vi "WUP.vi"() -> ()   [LabVIEW 2013]
uses:
  <userlib>/_OpenG.lib/array/array.llb/Index 1D Array Elements (String)__ogtk.vi
panel:
  in  "Experiment":u16(ring) items=["10TW", "test stand", "LaserUpstairs", "Staging"]
  out "clients dead":i16
  out "clients alive":i16
  in  "remote desktop":bool
  in  "Scrollbar":i32(c297)
  in  "cmd":bool
  out "Message 3":string
  in  "CMD":string
  out "error out 2":errorcluster
  in  "enter":bool
  out "elements":string[](array[string])
  in  "Listbox":i32[](listbox)
  out "output cluster":T1
  in  "ping":bool
  in  "WUP and restart":bool
  in  "stop":bool
  out "Message 2":string="\\\\192.168.10.217\\Documents\\Software\\LABVIEW\\Sven\\test\\wuInstall /search /criteria \"IsInstalled=0 and AutoSelectOnWebSites=1\""
  out "error out":errorcluster
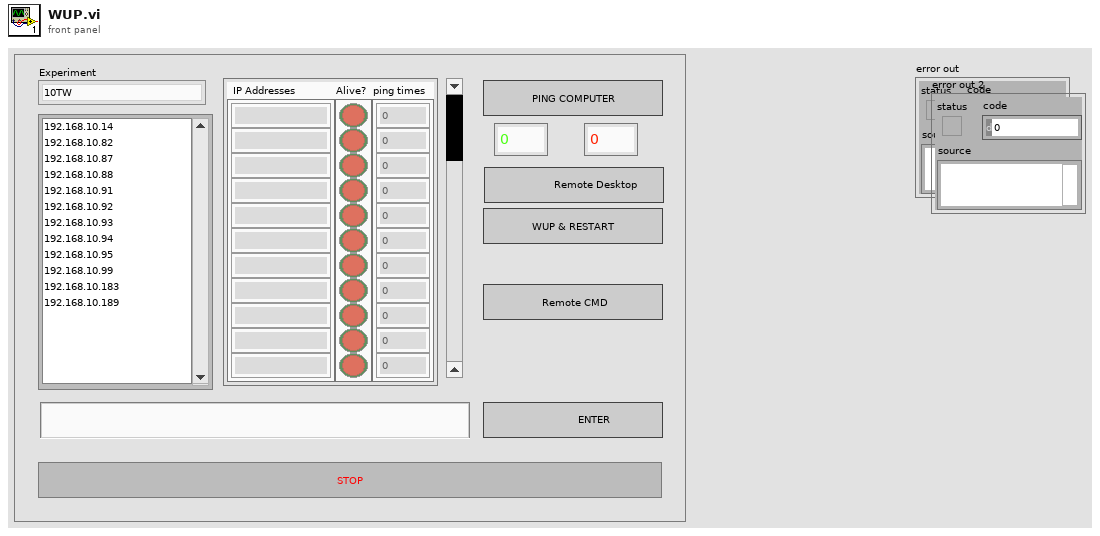
[diagram p1: front panel]
types:
  T1 = cluster{"IP Addresses ":string[], "Alive?":bool[], "ping times":u32[]}
  T2 = cluster{"elements":string[], "Awake?":bool[], "ping times [ms]":u32[]}
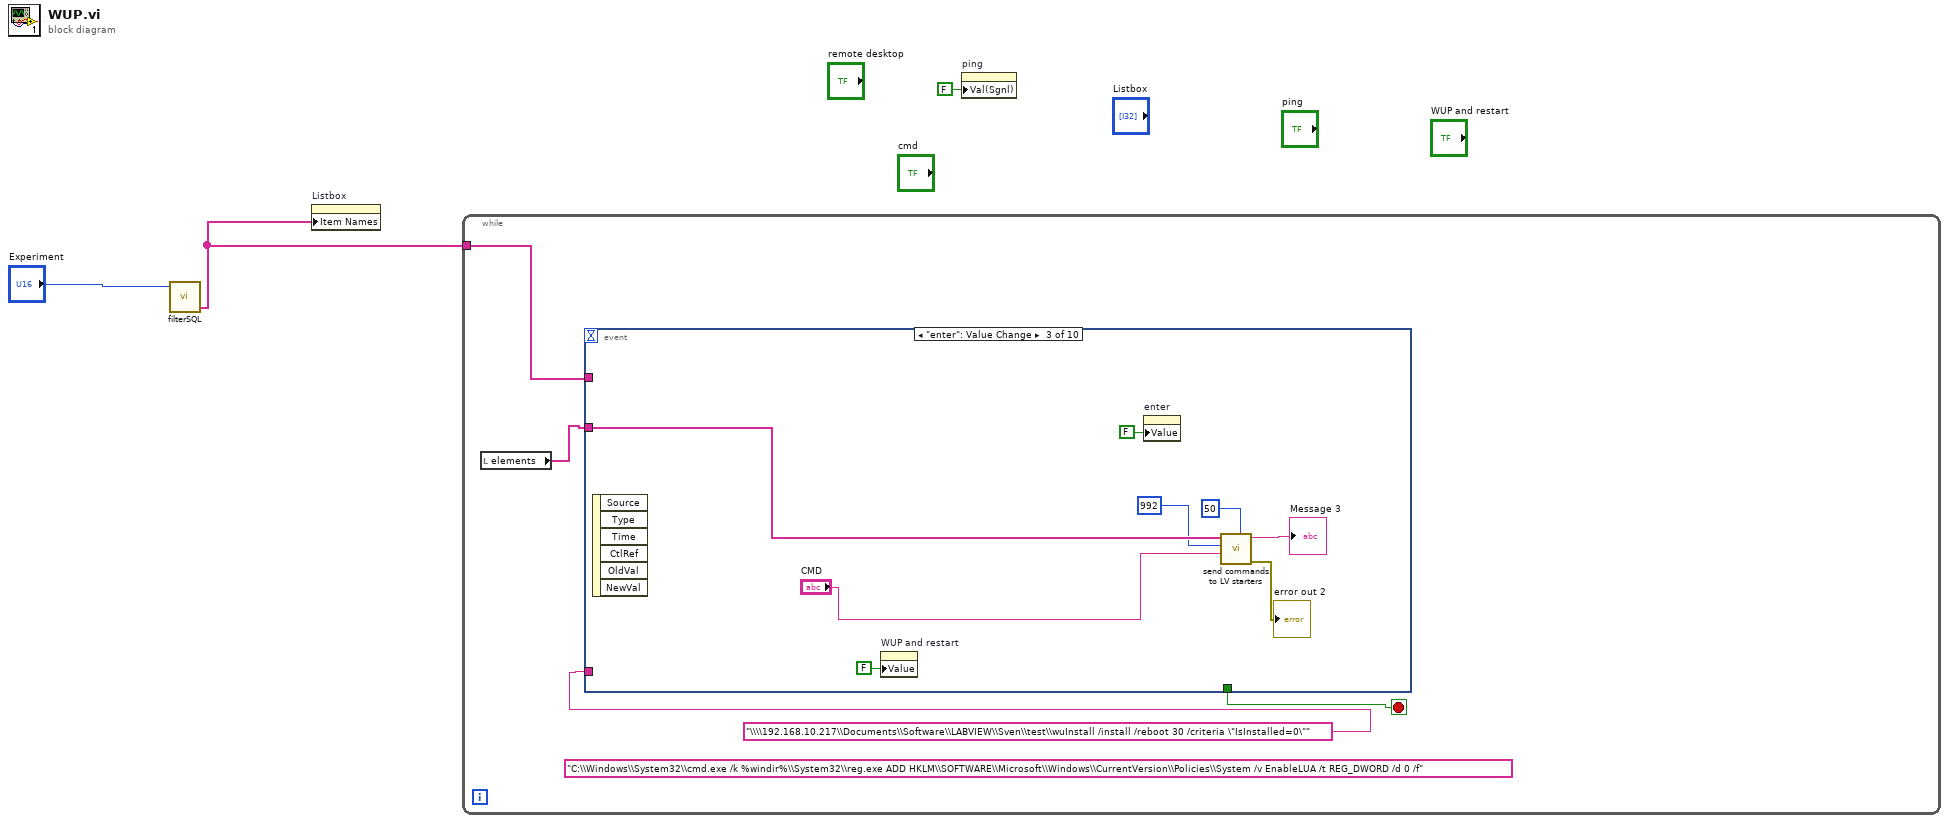
[diagram p0: block diagram]
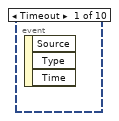
[diagram p2: hidden frame]
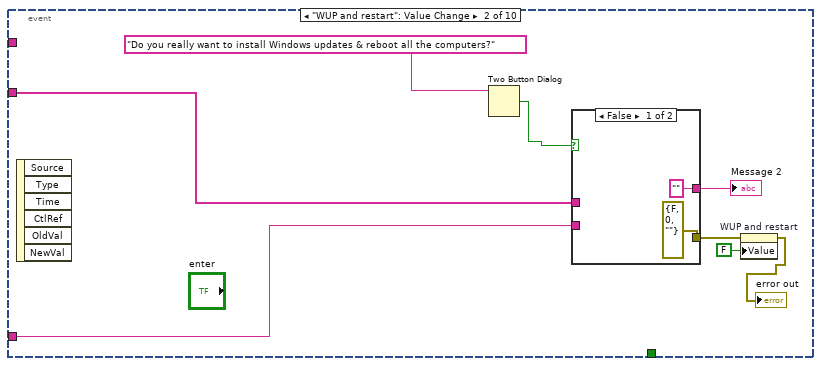
[diagram p3: hidden frame]
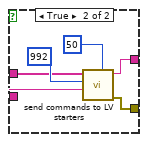
[diagram p4: hidden frame]
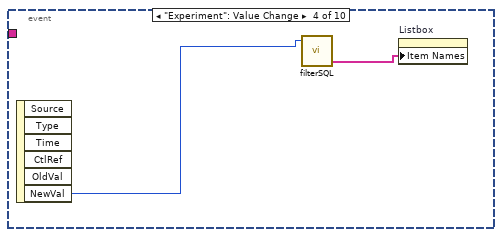
[diagram p5: hidden frame]
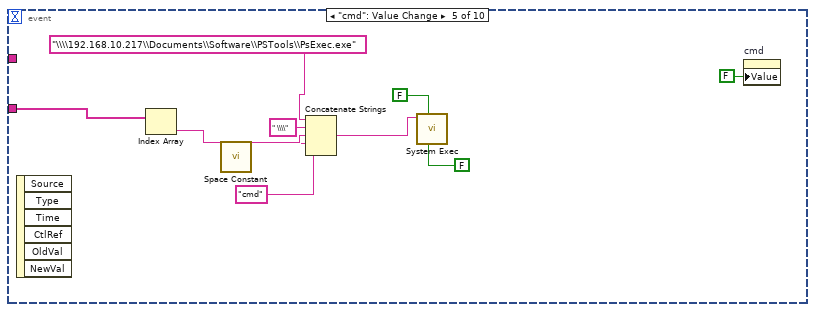
[diagram p6: hidden frame]
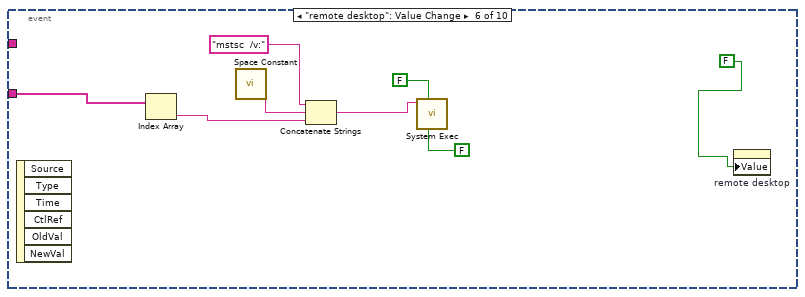
[diagram p7: hidden frame]
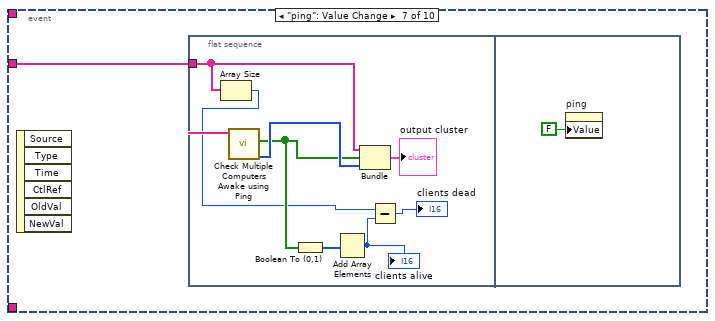
[diagram p8: hidden frame]
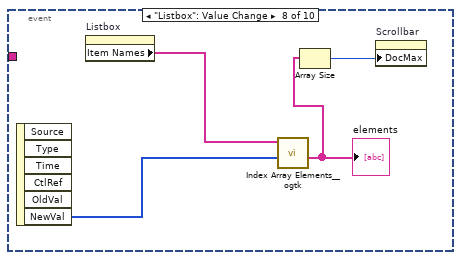
[diagram p9: hidden frame]
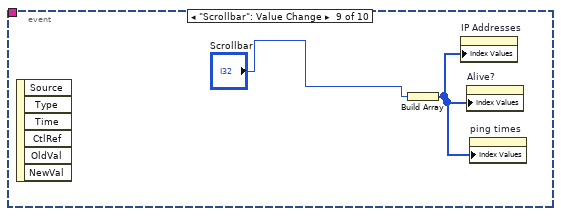
[diagram p10: hidden frame]
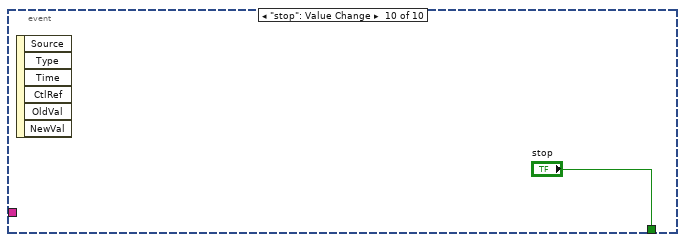
[diagram p11: hidden frame]
diagram:
  n1 = call "filterSQL.vi"("Experiment"="Experiment") -> ("filtered"=w1:string[])  [unwired: 3 in, 1 out]
  n2 = property on="Listbox" class="LstBox (strict)"("Item Names"=w1) -> ()  [unwired: 2 in, 2 out]
  n3 = while {
    tunnel: w1 -> [w6]
    stop <- w7 stop-if-true
    (unwired) "C:\\Windows\\System32\\cmd.exe /k %windir%\\System32\\reg.exe ADD HKLM\\SOFTWARE\\Microsoft\\Windows\\CurrentVersion\\Policies\\System /v EnableLUA /t REG_DWORD /d 0 /f"
    n4 = local read "elements"() -> (w4:string[])
    n5 = event shown="[2] \"enter\": Value Change" {
      selector: _ -> [_ _ _ _ _ _ _ _ _ _]
      dyn-events: _ -> [_ _ _ _ _ _ _ _ _ _]
      timeout: _ -> [_ _ _ _ _ _ _ _ _ _]
      tunnel: "\\\\192.168.10.217\\Documents\\Software\\LABVIEW\\Sven\\test\\wuInstall /install /reboot 30 /criteria \"IsInstalled=0\"" ("Message") -> [_ w15 _ _ _ _ _ _ _ _]
      tunnel: [_ _ _ _ _ _ _ _ _ "stop"] -> w7
      tunnel: w4 -> [_ w11 w30 _ w42 w51 w52 _ _ _]
      tunnel: w6 -> [_ _ _ _ _ _ _ _ _ _]
      event Timeout {
        n6 = event-data() -> ()  [unwired: 1 in, 3 out]
      }
      event "WUP and restart": Value Change {
        n7 = event-data() -> ()  [unwired: 1 in, 6 out]
        n8 = Two Button Dialog(message="Do you really want to install Windows updates & reboot all the computers?") -> (T button?=w12:bool)  [unwired: 2 in]
        n9 = case shown="False" w12 {
          tunnel: w11 -> [_ w21]
          tunnel: w15 -> [_ w20]
          tunnel: [errorcluster {"status"=FALSE, "code"=0, "source"=""} ("error out") w19] -> w10
          tunnel: ["" ("Message 2") w18] -> w8
          frame False {
          }
          frame True {
            n10 = call "send commands to LV starters.vi"("IP Addresses"=w21, "Local Port"=u16 992, "Message"=w20, "time between commands (ms)"=u32 50) -> ("Message 2"=w18:string, "error out"=w19:errorcluster)  [unwired: 4 in]
          }
        }
        "Message 2" <- w8
        n11 = property on="WUP and restart" class="Bool (strict)"(error in=w10, "Value"=FALSE ("WUP and restart")) -> (error out=→"error out":errorcluster)  [unwired: 1 in, 1 out]
      }
      event "enter": Value Change {
        n12 = event-data() -> ()  [unwired: 1 in, 6 out]
        n13 = property on="WUP and restart" class="Bool (strict)"("Value"=FALSE ("WUP and restart")) -> ()  [unwired: 2 in, 2 out]
        n14 = property on="enter" class="Bool (strict)"("Value"=FALSE ("enter")) -> ()  [unwired: 2 in, 2 out]
        n15 = call "send commands to LV starters.vi"("IP Addresses"=w30, "Local Port"=u16 992, "Message"="CMD", "time between commands (ms)"=u32 50) -> ("Message 2"=→"Message 3":string, "error out"=→"error out 2":errorcluster)  [unwired: 4 in]
      }
      event "Experiment": Value Change {
        n16 = event-data() -> ("NewVal"=w32:u16)  [unwired: 1 in, 5 out]
        n17 = call "filterSQL.vi"("Experiment"=w32) -> ("filtered"=w33:string[])  [unwired: 3 in, 1 out]
        n18 = property on="Listbox" class="LstBox (strict)"("Item Names"=w33) -> ()  [unwired: 2 in, 2 out]
      }
      event "cmd": Value Change {
        n19 = event-data() -> ()  [unwired: 1 in, 6 out]
        n20 = Index Array(array=w42) -> (element=w39:string)  [unwired: 1 in]
        n21 = call <vilib>:"Space Constant.vi"() -> ("String"=w35:string)
        n22 = Concatenate Strings("\\\\192.168.10.217\\Documents\\Software\\PSTools\\PsExec.exe" ("string"), " \\\\" ("string"), w39, w35, "cmd" ("string 2")) -> (w36:string)
        n23 = call <vilib>:"System Exec.vi"("run minimized? (F)"=FALSE, "wait until completion? (T)"=FALSE, "command line"=w36) -> ()  [unwired: 5 in, 4 out]
        n24 = property on="cmd" class="Bool (strict)"("Value"=FALSE ("New Button")) -> ()  [unwired: 2 in, 2 out]
      }
      event "remote desktop": Value Change {
        n25 = event-data() -> ()  [unwired: 1 in, 6 out]
        n26 = Index Array(array=w51) -> (element=w45:string)  [unwired: 1 in]
        n27 = call <vilib>:"Space Constant.vi"() -> ("String"=w46:string)
        n28 = Concatenate Strings("mstsc  /v:" ("string"), w46, w45) -> (w47:string)
        n29 = call <vilib>:"System Exec.vi"("run minimized? (F)"=FALSE, "wait until completion? (T)"=FALSE, "command line"=w47) -> ()  [unwired: 5 in, 4 out]
        n30 = property on="remote desktop" class="Bool (strict)"("Value"=FALSE ("New Button")) -> ()  [unwired: 2 in, 2 out]
      }
      event "ping": Value Change {
        n31 = event-data() -> ()  [unwired: 1 in, 6 out]
        n32 = flat-sequence {
          tunnel: w52 -> [w56]
          frame #0 {
            n33 = Array Size(array=w56) -> (size(s)=w55:i32)
            n34 = call "Check Multiple Computers Awake using Ping.vi"("List of IPs"=w56) -> ("ping times [ms]"=w60:u32[], "Awake?"=w58:bool[])  [unwired: 8 in, 1 out]
            n35 = Boolean To (0,1)(Boolean=w58) -> (0, 1=w57:i16[])
            n36 = Add Array Elements(numeric array=w57) -> (sum=w54:i16)
            "clients alive" <- w54
            n37 = Bundle("elements"=w56, "Awake?"=w58, "ping times [ms]"=w60) -> (→"output cluster":T2)  [unwired: 1 in]
            n38 = Subtract(x=w55, y=w54) -> (x-y=→"clients dead":i32)
          }
          frame #1 {
            n39 = property on="ping" class="Bool (strict)"("Value"=FALSE ("ping")) -> ()  [unwired: 2 in, 2 out]
          }
        }
      }
      event "Listbox": Value Change {
        n40 = event-data() -> ("NewVal"=w65:i32[])  [unwired: 1 in, 5 out]
        n41 = property on="Listbox" class="LstBox (strict)"() -> ("Item Names"=w62:string[])  [unwired: 2 in, 2 out]
        n42 = call-poly <userlib>:"Index Array Elements__ogtk.vi"("indices"=w65, "array"=w62) -> ("elements"=w63:string[])  [unwired: 9 in]
        "elements" <- w63
        n43 = Array Size(array=w63) -> (size(s)=w64:i32)
        n44 = property on="Scrollbar" class="Scroll (strict)"("DocMax"=w64) -> ()  [unwired: 2 in, 2 out]
      }
      event "Scrollbar": Value Change {
        n45 = event-data() -> ()  [unwired: 1 in, 6 out]
        n46 = Build Array("Scrollbar") -> (w66:i32[])
        n47 = property on="IP Addresses" class="Arr (strict)"("Index Values"=w66) -> ()  [unwired: 2 in, 2 out]
        n48 = property on="Alive?" class="Arr (strict)"("Index Values"=w66) -> ()  [unwired: 2 in, 2 out]
        n49 = property on="ping times" class="Arr (strict)"("Index Values"=w66) -> ()  [unwired: 2 in, 2 out]
      }
      event "stop": Value Change {
        n50 = event-data() -> ()  [unwired: 1 in, 6 out]
      }
    }
  }
  n51 = property on="ping" class="Bool (strict)"("Val(Sgnl)"=FALSE ("Value (Signaling)")) -> ()  [unwired: 2 in, 2 out]
